vi "tag select action.vi"(8 "engine":refnum<data-value>, 10 "CtlRef":refnum<vi>, 11 "module editor":refnum<data-value>) -> (0 "error out":errorcluster)   [LabVIEW 2013]
uses:
  <vilib>/NI/Tag Bus/tag/tag descriptor.lvclass
  <vilib>/NI/Configuration Framework/serializable configuration/NISE_CEF_serializable configuration.lvclass
  <vilib>/NI/Tag Bus Data Framework/Configuration Editor/Classes/Engine Parent/Engine Parent Editor Node.lvclass
  <vilib>/NI/Module Execution Interface/Engine Configuration/engine configuration.lvclass
  <vilib>/NI/Tag Bus Data Framework/control module/configuration/control module configuration.lvclass
  <vilib>/NI/Tag Bus Data Framework/control module/editor node/control module editor.lvclass
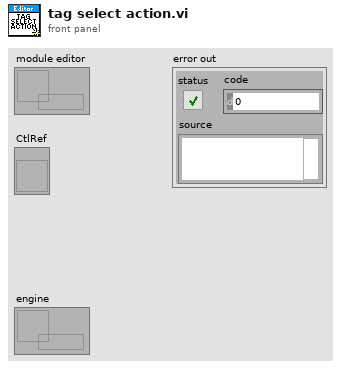
[diagram p1: front panel]
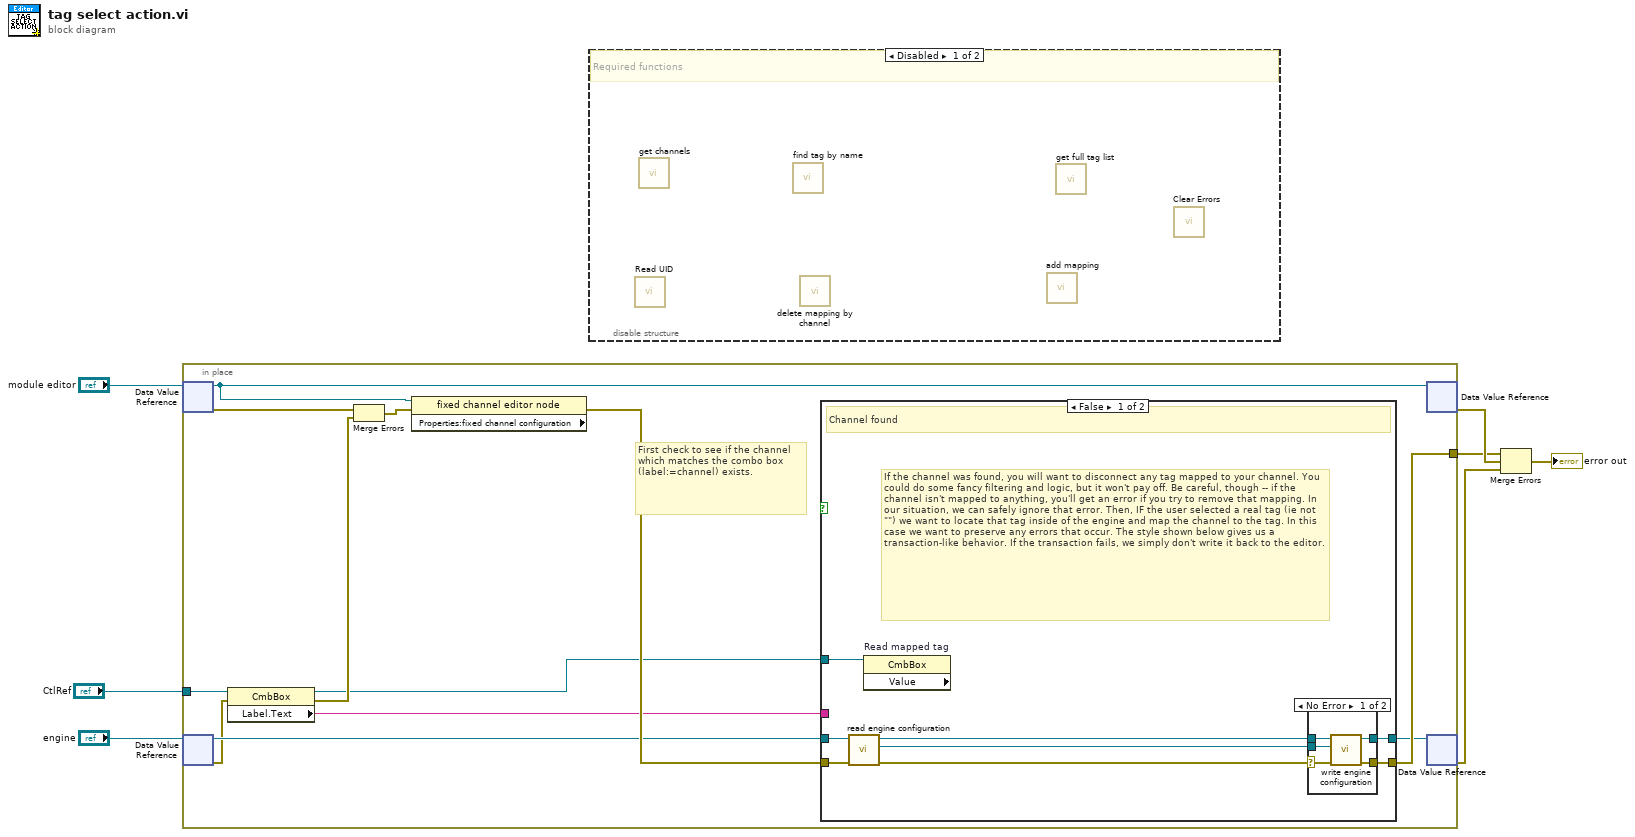
[diagram p0: block diagram]
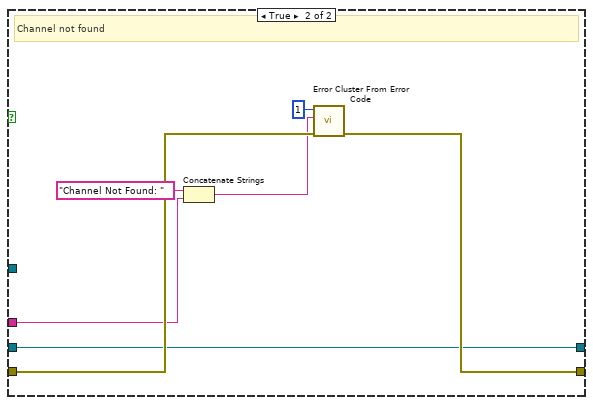
[diagram p4: hidden frame]
diagram:
  n1 = in-place {
    in-place-border: [w18] -> w2
    in-place-border: "CtlRef" -> [w16]
    # "First check to see if the channel which matches the combo box (label:=channel) exists."
    n2 = in-place-dvr #1("module editor") -> (w14:refnum<class "control module editor.lvclass">, w19:errorcluster)
    n3 = in-place-dvr #2("engine") -> (w13:refnum<class "Engine Parent Editor Node.lvclass">, w10:errorcluster)
    n4 = property class="CmbBox"(reference=w16, error in=w10) -> (reference out=w8:refnum<vi>, error out=w11:errorcluster, "Label.Text"=w9:string)
    n5 = Merge Errors(w19, w11) -> (w15:errorcluster)
    n6 = property class="fixed channel editor node" props=["Properties:fixed channel configuration"](reference=w14, error in=w15) -> (error out=w17:errorcluster)  [unwired: 2 out]
    n7 = case shown="False" {
      selector: _ -> [_ _]
      tunnel: [w25 w40] -> w18
      tunnel: w17 -> [w23 w39]
      tunnel: w13 -> [w27 w38]
      tunnel: [w26 w38] -> w12
      tunnel: w9 -> [_ w35]
      tunnel: w8 -> [w20 _]
      frame False {
        # "If the channel was found, you will want to disconnect any tag mapped to your channel. You could do some fancy filtering and logic, but it won't pay off. Be careful, though -- if the channel isn't mapped to anything, you'll get an error if you try to remove that mapping. In our situation, we can safely ignore that error. Then, IF the user selected a real tag (ie not \"\") we want to locate that tag inside of the engine and map the channel to the tag. In this case we want to preserve any errors that occur. The style shown below gives us a transaction-like behavior. If the transaction fails, we simply don't write it back to the editor."
        # "Channel found"
        n8 = call <vilib>:"read engine configuration.vi"("error in"=w23, "Engine Parent Editor Node in"=w27) -> ("error out"=w22:errorcluster, "engine configuration"=w21:refnum<class "engine configuration.lvclass">, "Engine Parent Editor Node out"=w24:refnum<class "Engine Parent Editor Node.lvclass">)  [unwired: 7 in]
        n9 = property on="Read mapped tag" class="CmbBox" props=["Value"](reference=w20) -> ()  [unwired: 1 in, 3 out]
        n10 = case shown="No Error" w22 {
          selector: w22 -> [w31 w33]
          tunnel: [w32 w34] -> w26
          tunnel: [w30 w33] -> w25
          tunnel: w24 -> [w29 w34]
          tunnel: w21 -> [w28 _]
          frame No Error {
            n11 = call <vilib>:"write engine configuration.vi"("error in"=w31, "engine configuration"=w28, "Engine Parent Editor Node in"=w29) -> ("error out"=w30:errorcluster, "Engine Parent Editor Node out"=w32:refnum<class "Engine Parent Editor Node.lvclass">)  [unwired: 7 in]
          }
          frame Error {
          }
        }
      }
      frame True {
        # "Channel not found"
        n12 = Concatenate Strings("Channel Not Found: " ("string"), w35) -> (w37:string)
        n13 = call <vilib>:"Error Cluster From Error Code.vi"("error in (no error)"=w39, "error message (\"\")"=w37, "error code (0)"=1) -> ("error out"=w40:errorcluster)  [unwired: 6 in]
      }
    }
    n14 = in-place-dvr #1(w14) -> (w3:errorcluster)  [unwired: 1 out]
    n15 = in-place-dvr #2(w12) -> (w6:errorcluster)  [unwired: 1 out]
  }
  n16 = disable-structure shown="Disabled" {
    frame Disabled {
      # "Required functions"
      n17 = call <vilib>:"Read UID.vi"() -> ()  [unwired: 9 in, 3 out]
      n18 = call-dynamic "get channels.vi"() -> ()  [unwired: 10 in, 2 out]
      n19 = call <vilib>:"find tag by name.vi"() -> ()  [unwired: 11 in, 1 out]
      n20 = call <vilib>:"delete mapping by channel.vi"() -> ()  [unwired: 10 in, 2 out]
      n21 = call <vilib>:"add mapping.vi"() -> ()  [unwired: 10 in, 2 out]
      n22 = call <vilib>:"get full tag list.vi"() -> ()  [unwired: 10 in, 2 out]
      n23 = call <vilib>:"Clear Errors.vi"() -> ()  [unwired: 6 in, 2 out]
    }
    frame Enabled {
    }
  }
  n24 = Merge Errors(w2, w3, w6) -> (→"error out":errorcluster)
